vi "odczytywanie.vi"() -> ()   [LabVIEW 2020]
uses:
  <vilib>/Utility/xml.llb/Write to XML File(string).vi
panel:
  out "bytes written":i32
  out "xml string":string
  out "path":path
  in  "Stop Button":bool
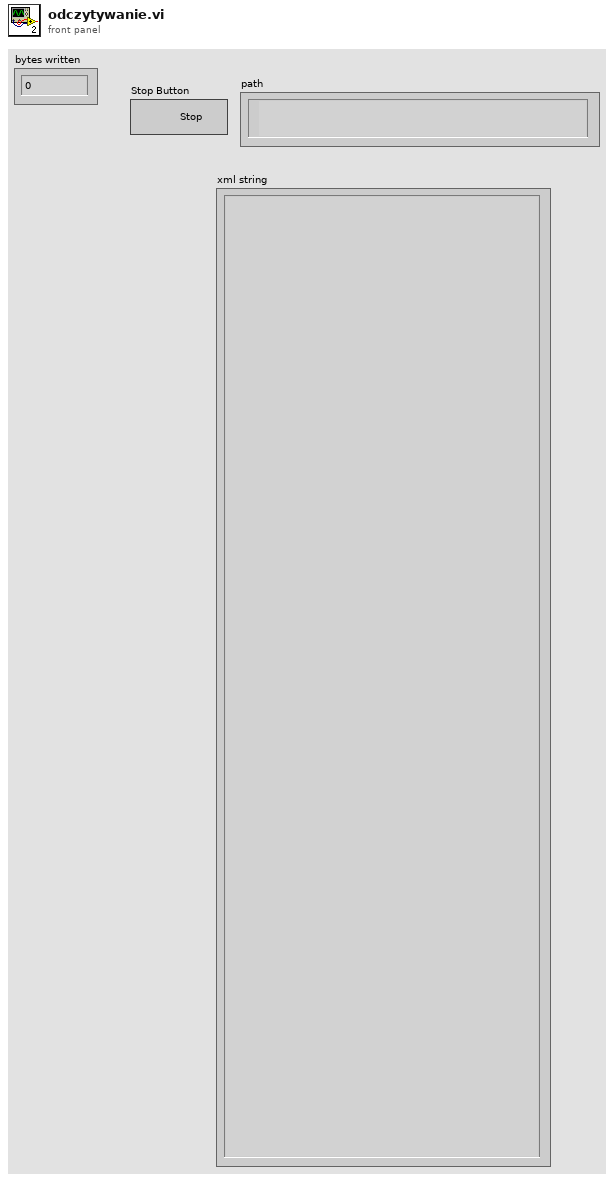
[diagram p1: front panel]
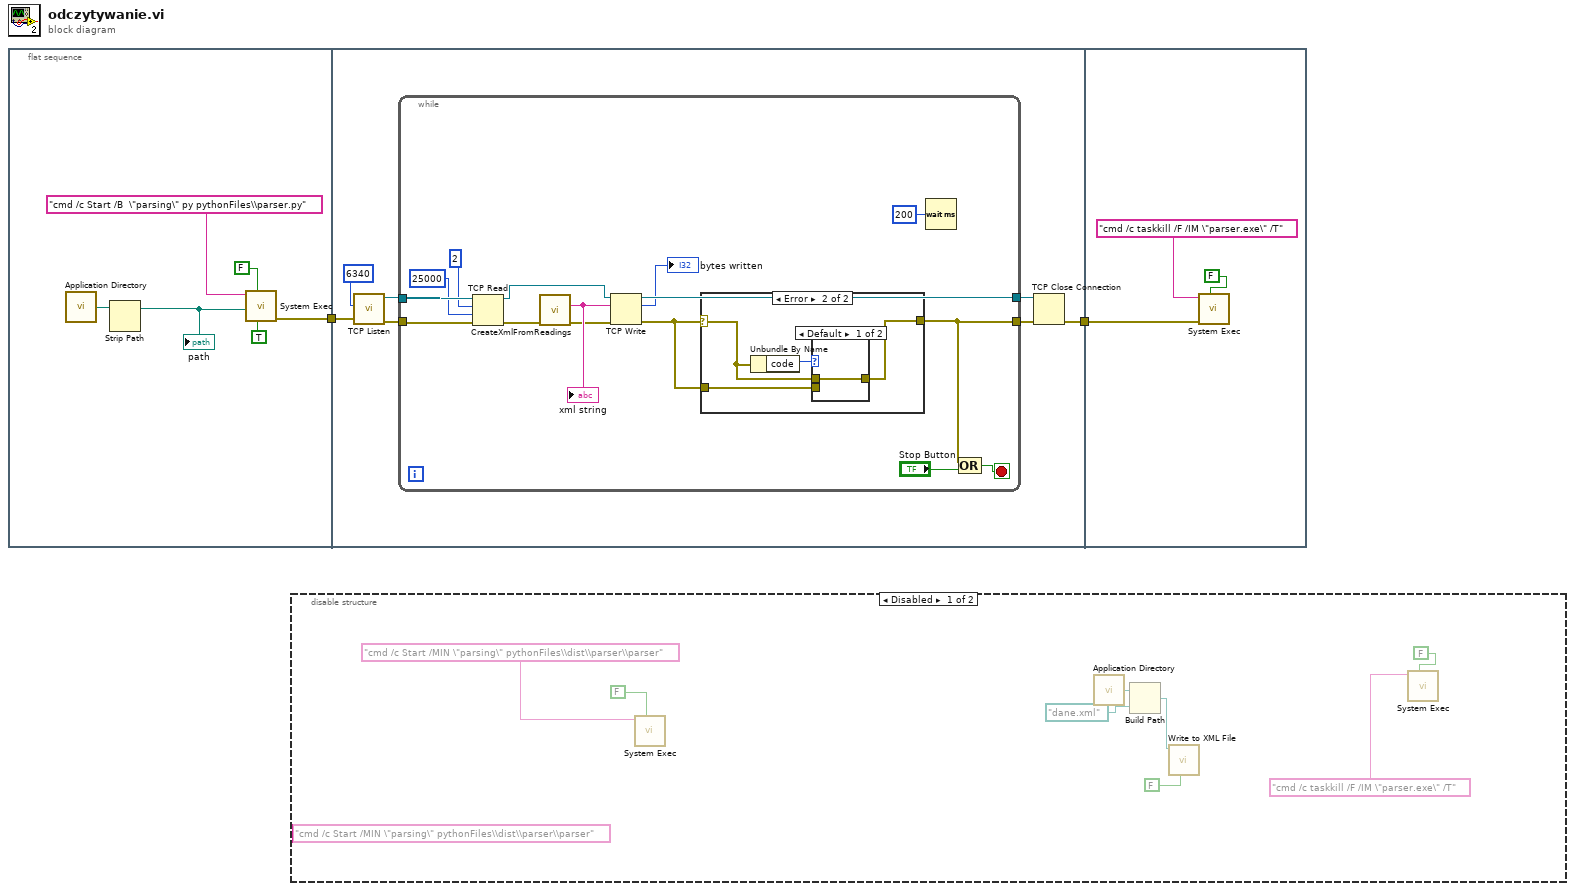
[diagram p0: block diagram]
diagram:
  n1 = flat-sequence {
    tunnel: [w7] -> w2
    tunnel: w2 -> [w12]
    tunnel: [w9] -> w1
    tunnel: w1 -> [w38]
    frame #0 {
      n2 = call <vilib>:"Application Directory.vi"() -> ("Application Directory"=w4:path)
      n3 = Strip Path(path=w4) -> (stripped path=w3:path)  [unwired: 1 out]
      "path" <- w3
      n4 = call <vilib>:"System Exec.vi"("run minimized? (F)"=TRUE, "wait until completion? (T)"=FALSE, "working directory"=w3, "command line"="cmd /c Start /B  \"parsing\" py pythonFiles\\parser.py") -> ("error out"=w7:errorcluster)  [unwired: 4 in, 3 out]
    }
    frame #1 {
      n5 = call <vilib>:"TCP Listen.vi"("error in (no error)"=w12, "port"=u16 6340) -> ("error out"=w11:errorcluster, "connection ID"=w14:refnum<k5>)  [unwired: 5 in, 3 out]
      n6 = while {
        tunnel: w14 -> [w28]
        tunnel: [w30] -> w13
        tunnel: w11 -> [w23]
        tunnel: [w20] -> w10
        stop <- w21 stop-if-true
        n7 = TCP Read(connection ID=w28, bytes to read=2, error in (no error)=w23, 9:25000 ("timeout ms (25000)")) -> (connection ID out=w27:refnum<k5>, error out=w18:errorcluster)  [unwired: 1 in, 1 out]
        n8 = call "CreateXmlFromReadings.vi"("error in"=w18) -> ("error out"=w17:errorcluster, "xml string"=w24:string)  [unwired: 9 in]
        "xml string" <- w24
        n9 = TCP Write(connection ID=w27, data in=w24, error in (no error)=w17) -> (connection ID out=w30:refnum<k5>, bytes written=→"bytes written":i32, error out=w19:errorcluster)  [unwired: 1 in]
        n10 = case shown="Error" w19 {
          selector: w19 -> [w31 w33]
          tunnel: [w31 w34] -> w20
          tunnel: w19 -> [_ w32]
          frame No Error {
          }
          frame Error {
            n11 = Unbundle By Name(w33) -> ("code"=w35:i32)
            n12 = case shown="Default" w35 {
              tunnel: w33 -> [w36 _]
              tunnel: w32 -> [_ w37]
              tunnel: [w36 w37] -> w34
              frame Default {
              }
              frame 56 {
              }
            }
          }
        }
        n13 = Wait (ms)(milliseconds to wait=u32 200) -> ()  [unwired: 1 out]
        n14 = Compound Arithmetic op=OR(w20, "Stop Button") -> (w21:bool)
      }
      n15 = TCP Close Connection(connection ID=w13, error in (no error)=w10) -> (error out=w9:errorcluster)  [unwired: 1 in, 1 out]
    }
    frame #2 {
      n16 = call <vilib>:"System Exec.vi"("wait until completion? (T)"=FALSE, "error in (no error)"=w38, "command line"="cmd /c taskkill /F /IM \"parser.exe\" /T") -> ()  [unwired: 5 in, 4 out]
    }
  }
  n17 = disable-structure shown="Disabled" {
    frame Disabled {
      (unwired) "cmd /c Start /MIN \"parsing\" pythonFiles\\dist\\parser\\parser" ("command line")
      n18 = call <vilib>:"System Exec.vi"("wait until completion? (T)"=FALSE, "command line"="cmd /c Start /MIN \"parsing\" pythonFiles\\dist\\parser\\parser") -> ()  [unwired: 6 in, 4 out]
      n19 = call <vilib>:"Application Directory.vi"() -> ("Application Directory"=w47:path)
      n20 = Build Path(base path=w47, name or relative path=path "dane.xml" ("File Path")) -> (appended path=w48:path)
      n21 = call-poly <vilib>:"Write to XML File.vi"("Standalone? (T)"=FALSE, "XML File Path"=w48) -> ()  [unwired: 7 in, 3 out]
      n22 = call <vilib>:"System Exec.vi"("wait until completion? (T)"=FALSE, "command line"="cmd /c taskkill /F /IM \"parser.exe\" /T") -> ()  [unwired: 6 in, 4 out]
    }
    frame Enabled {
    }
  }
